vi "Read Settings.vi"(8 "error in (no error)":errorcluster, 11 "LakeShore 340 in":refnum<class "LakeShore 340.lvclass">) -> (0 "error out":errorcluster, 2 "Settings":string, 3 "LakeShore 340 out":refnum<class "LakeShore 340.lvclass">)   [LabVIEW 2015, in "LakeShore 340.lvclass"]
uses:
  LakeShore 340.lvclass
  Instrument/Instrument.lvclass
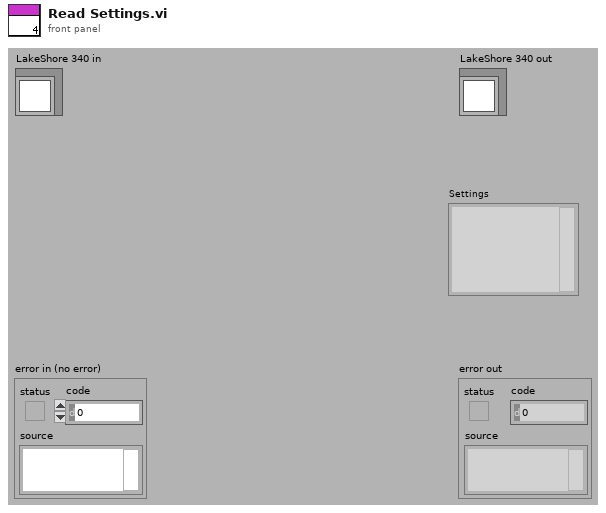
[diagram p1: front panel]
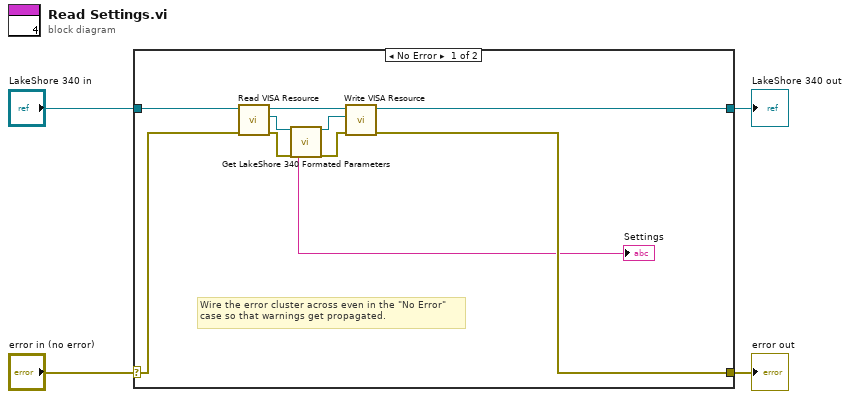
[diagram p0: block diagram]
diagram:
  n1 = case shown="No Error" "error in (no error)" {
    selector: "error in (no error)" -> [w9 w16]
    tunnel: [w6 w16] -> w3
    tunnel: [w11 w15] -> w1
    tunnel: "LakeShore 340 in" -> [w14 w15]
    frame No Error {
      # "Wire the error cluster across even in the \"No Error\"\ncase so that warnings get propagated."
      n2 = call "Read VISA Resource.vi"("error in (no error)"=w9, "Instrument.lvclass in"=w14) -> ("error out"=w8:errorcluster, "VISA Resource"=w12:refnum<visa-resource-name>, "Instrument.lvclass out"=w13:refnum<class "LakeShore 340.lvclass">)  [unwired: 7 out]
      n3 = call "Get LakeShore 340 Formated Parameters.vi"("VISA Resource Name"=w12, "error in (no error)"=w8) -> ("Parameters"=→"Settings":string, "VISA Resource Name Out"=w10:refnum<visa-resource-name>, "error out"=w7:errorcluster)  [unwired: 1 in, 14 out]
      n4 = call "Write VISA Resource.vi"("error in (no error)"=w7, "VISA Resource"=w10, "Instrument.lvclass in"=w13) -> ("error out"=w6:errorcluster, "Instrument.lvclass out"=w11:refnum<class "LakeShore 340.lvclass">)  [unwired: 7 out]
    }
    frame Error {
    }
  }
  "error out" <- w3
  "LakeShore 340 out" <- w1
